vi "Read Notifier.vi"(11 "TestManagerMsg.CompleteSuite in":refnum<class "TestManagerMsg.CompleteSuite.lvclass">) -> (2 "notifier":refnum<notifier>, 3 "TestManagerMsg.CompleteSuite out":refnum<class "TestManagerMsg.CompleteSuite.lvclass">)   [LabVIEW 2013, in "Caraya.lvlib" / "TestManagerMsg.CompleteSuite.lvclass"]
uses:
  TestManagerMsg.CompleteSuite.lvclass
  TestManagerMsg.CompleteSuite.lvclass/TestManagerMsg.CompleteSuite.ctl
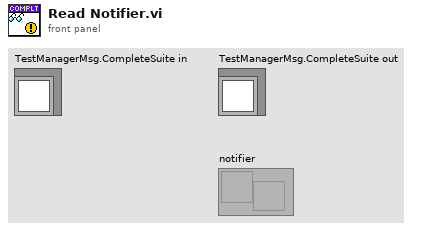
[diagram p1: front panel]
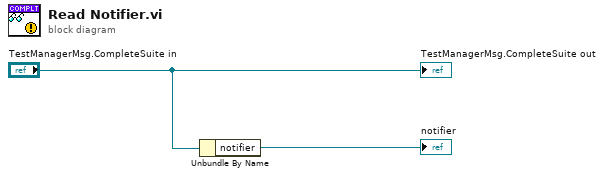
[diagram p0: block diagram]
diagram:
  n1 = Unbundle By Name("TestManagerMsg.CompleteSuite in") -> ("notifier"=→"notifier":refnum<notifier>)
  "TestManagerMsg.CompleteSuite out" <- "TestManagerMsg.CompleteSuite in"
